vi "Keithley2450_and_2410_plus_lockin.vi"() -> ()   [LabVIEW 2024]
uses:
  <vilib>/Analysis/1siggen.llb/Ramp Pattern by Delta.vi
  <vilib>/Utility/file.llb/Write Delimited Spreadsheet (string).vi
  <vilib>/Utility/file.llb/Write Delimited Spreadsheet (DBL).vi
  C:/Users/Public/OneDrive/Desktop/Keithley_2450_2470_1_4_0_LV2015_NewReadme2_2450-LV2015-1.4.0/Keithley 2450/Keithley 2450.lvlib
  <vilib>/Analysis/NI_AALBase.lvlib
  archive/Keithley 24XX/Keithley 24XX.lvlib
panel:
  out "voltage 2410":dbl format="%0.2f"
  out "Current set voltage 2410":dbl
  in  "V stepsize 2410":dbl
  in  "start V 2410":dbl
  in  "End V 2410":dbl
  out "standard deviation current measured 2450":dbl format="%0.5e"
  out "mean current measured 2450":dbl format="%0.5e"
  out "standard deviation current measured 2410":dbl format="%0.5e"
  out "mean current measured 2410":dbl format="%0.5e"
  in  "Compliance  Level 2410":dbl=1e-06
  in  "VISA resource name 2410":refnum<visa-resource-name>="GPIB0::24::INSTR"
  in  "Serial Configuration":T1={"Baud Rate"=9600, "Parity"=0, "Data Bits"=8, "Stop Bits"=10, "Flow Control"=0} {"Flow Control" items=["None", "XON/XOFF", "RTS/CTS", "XON/XOFF & RTS/CTS", "DTR/DSR", "XON/XOFF & DTR/DSR"]; "Stop Bits" items=["1.0"=10, "1.5"=15, "2.0"=20]; "Data Bits" items=["7"=7, "8"=8]; "Parity" items=["None", "Odd", "Even", "Mark", "Space"]; "Baud Rate" items=["300"=300, "600"=600, "1200"=1200, "2400"=2400, "4800"=4800, "9600"=9600, "19200"=19200]}
  in  "Wait for Current Meas":u32=100
  in  "Number of Current Meas":u32=100
  in  "Loop?":bool=TRUE
  out "Current set voltage 2450":dbl
  in  "V stepsize 2450":dbl
  in  "start V 2450":dbl
  in  "End V 2450":dbl
  in  "Wait for lock in meas (ms)":i32=2000
  in  "File Path":path=path "C:/Users/Public/OneDrive/Desktop/test.txt"
  out "错误输出":errorcluster
  out "Channel AWaveform Chart":dbl[](graph)
  in  "Channel A Waveform Display":string(combo)="A-R"
  in  "Channel B Waveform Display":string(combo)="Channel_B_Rh1"
  out "Channel B Waveform Chart":dbl[](graph)
  out "AUX-ADC4 (V)":sgl format="%.3f"
  out "AUX-ADC3 (V)":sgl format="%.3f"
  out "AUX-ADC1 (V)":sgl format="%.3f"
  out "AUX-ADC2 (V)":sgl format="%.3f"
  out "R":sgl caption="R (Vrms)" format="%.3p"
  out "X":sgl caption="X (Vrms)" format="%.3p"
  out "Y":sgl caption="Y (Vrms)" format="%.3p"
  out "θ (°)":sgl caption="θ (deg)" format="%.2f"
  out "频率 (Hz)":sgl caption="Freq (Hz)" format="%#.3f"
  out "噪声":sgl caption="Noise(Vrms)" format="%.3p"
  out "Rh1":sgl caption="Rh1 (Vrms)" format="%.3p"
  out "θh1 (°)":sgl caption="θh1 (deg)" format="%.2f"
  out "Xh1":sgl caption="Xh1 (Vrms)" format="%.3p"
  out "Yh1":sgl caption="Yh1 (Vrms)" format="%.3p"
  out "X 2":sgl caption="X (Vrms)" format="%.3p"
  out "Y 2":sgl caption="Y (Vrms)" format="%.3p"
  out "R 2":sgl caption="R (Vrms)" format="%.3p"
  out "θ (°) 2":sgl caption="θ (deg)" format="%.2f"
  out "频率 (Hz) 2":sgl caption="Freq (Hz)" format="%#.3f"
  out "噪声 2":sgl caption="Noise(Vrms)" format="%.3p"
  out "Xh1 2":sgl caption="Xh1 (Vrms)" format="%.3p"
  out "Yh1 2":sgl caption="Yh1 (Vrms)" format="%.3p"
  out "Rh1 2":sgl caption="Rh1 (Vrms)" format="%.3p"
  out "θh1 (°) 2":sgl caption="θh1 (deg)" format="%.2f"
  in  "A Sensitivity":u16(ring)=20 items=["1 nV/fA", "2 nV/fA", "5 nV/fA", "10 nV/fA", "20 nV/fA", "50 nV/fA", "100 nV/fA", "200 nV/fA", "500 nV/fA", "1 uV/pA", "2 uV/pA", "5 uV/pA", "10 uV/pA", "20 uV/pA", "50 uV/pA", "100 uV/pA", "200 uV/pA", "500 uV/pA", "1 mV/nA", "2 mV/nA", "5 mV/nA", "10 mV/nA", "20 mV/nA", "50 mV/nA", "100 mV/nA", "200 mV/nA", "500 mV/nA", "1 V/uA"]
  in  "B Sensitivity":u16(ring)=17 items=["1 nV/fA", "2 nV/fA", "5 nV/fA", "10 nV/fA", "20 nV/fA", "50 nV/fA", "100 nV/fA", "200 nV/fA", "500 nV/fA", "1 uV/pA", "2 uV/pA", "5 uV/pA", "10 uV/pA", "20 uV/pA", "50 uV/pA", "100 uV/pA", "200 uV/pA", "500 uV/pA", "1 mV/nA", "2 mV/nA", "5 mV/nA", "10 mV/nA", "20 mV/nA", "50 mV/nA", "100 mV/nA", "200 mV/nA", "500 mV/nA", "1 V/uA"]
  out "序列号":string
  in  "Num Lock in Points":i32=100
  in  "OE1022D":refnum<visa-resource-name>="COM6"
  in  "Current Compliance Limit (0.1) 2450":dbl=5e-08
  in  "VISA resource name 2450":refnum<visa-resource-name>="GPIB0::18::INSTR"
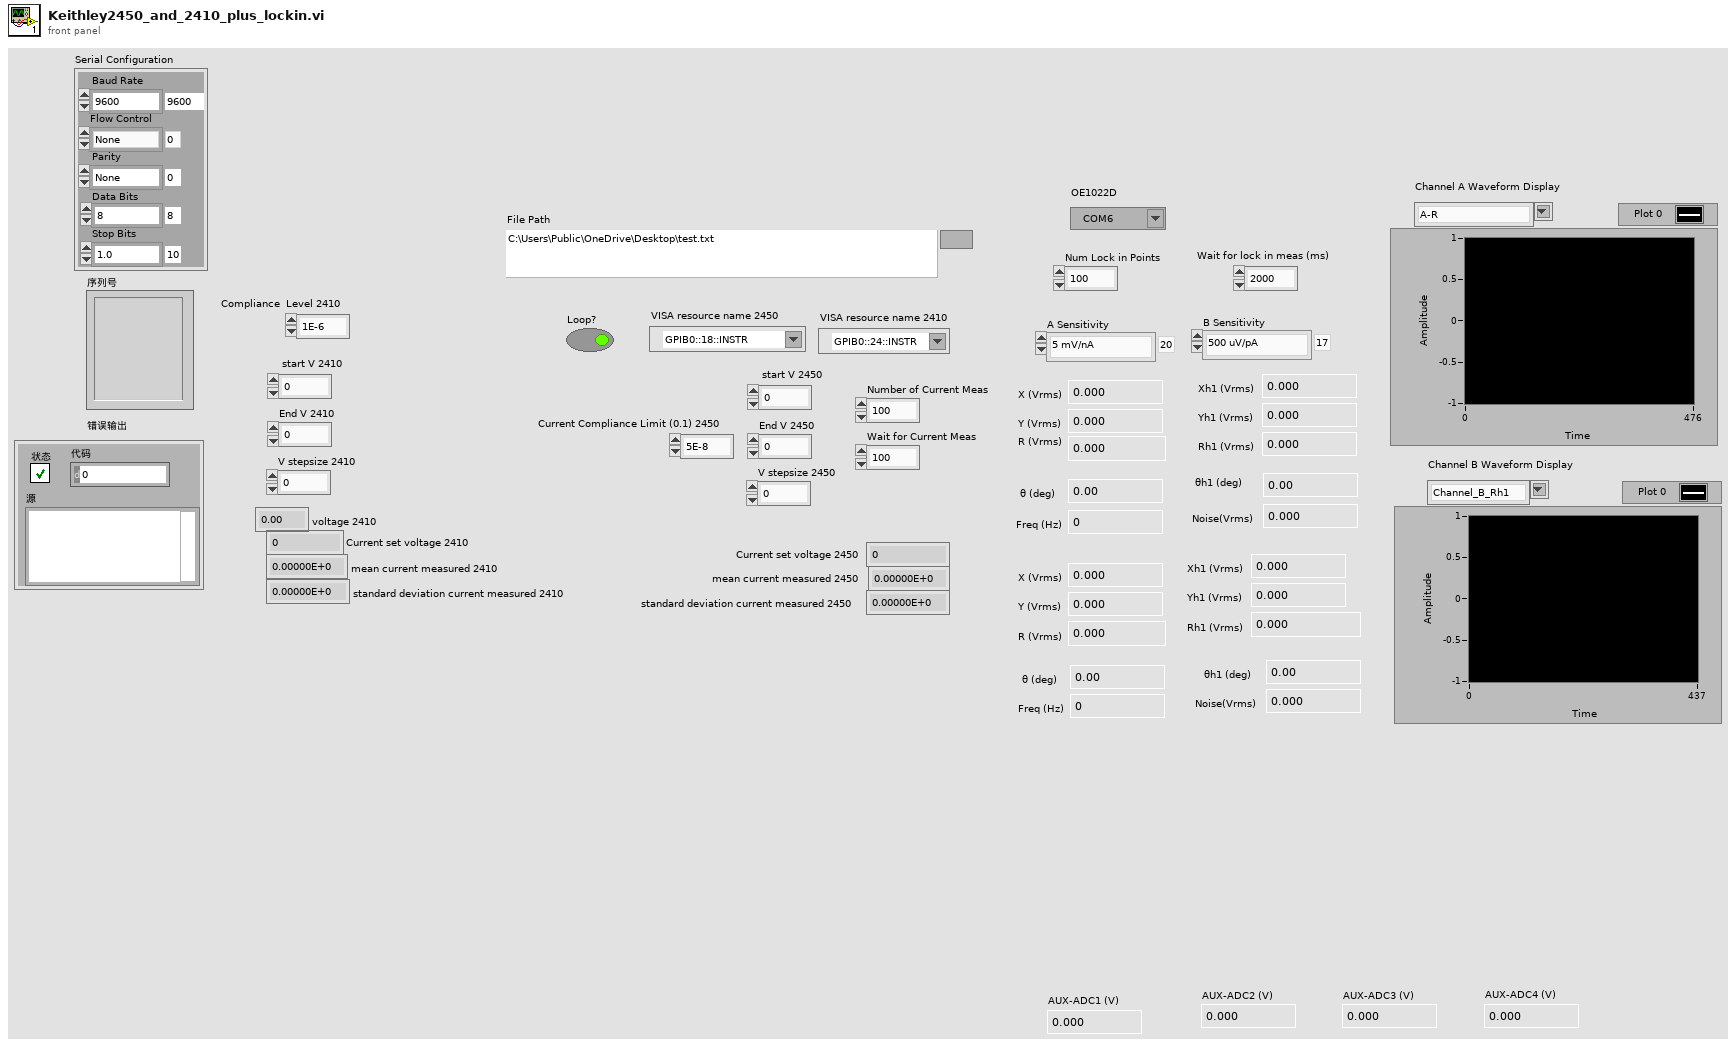
[diagram p1: front panel]
types:
  T1 = cluster{"Baud Rate":u32, "Parity":u16, "Data Bits":u16, "Stop Bits":u16, "Flow Control":u16}
  T2 = cluster{"AD1":dbl[], "AD2":dbl[], "AD3":dbl[], "AD4":dbl[]}
  T3 = cluster{"XB":dbl[], "YB":dbl[], "FrequencyB":dbl[], "NoiseB":dbl[], "Xh1B":dbl[], "Yh1B":dbl[], "Xh2B":dbl[], "Yh2B":dbl[], "Xh2B":dbl[]}
  T4 = cluster{"XA":dbl[], "YA":dbl[], "FrequencyA":dbl[], "NoiseA":dbl[], "Xh1A":dbl[], "Yh1A":dbl[], "Xh2A":dbl[], "Yh2A":dbl[]}
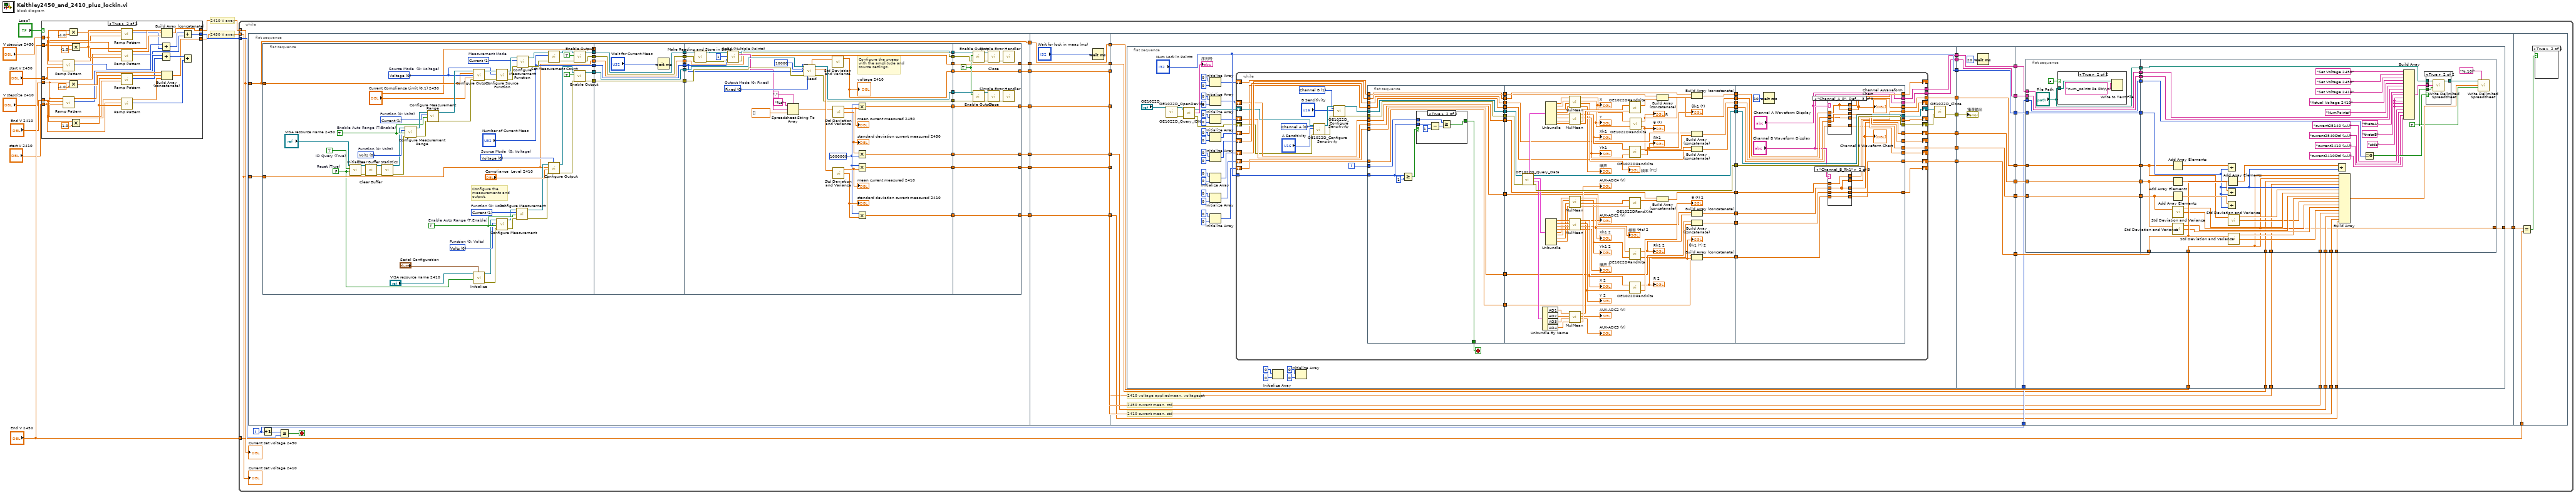
[diagram p0: block diagram]
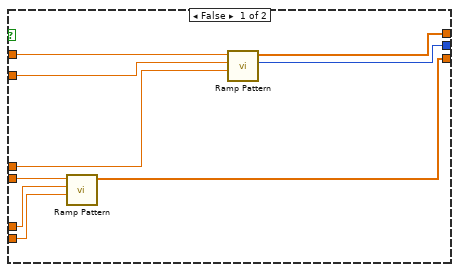
[diagram p2: hidden frame]
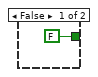
[diagram p3: hidden frame]
diagram:
  # "2410 V array"
  # "2450 V array"
  n1 = case shown="True" "Loop?" {
    tunnel: [w16 w43] -> w10
    tunnel: [w15 w38] -> w9
    tunnel: "V stepsize 2450" -> [w17 w37]
    tunnel: "start V 2450" -> [w18 w36]
    tunnel: "End V 2450" -> [w19 w35]
    tunnel: "End V 2410" -> [w14 w23]
    tunnel: "V stepsize 2410" -> [w12 w21]
    tunnel: "start V 2410" -> [w13 w22]
    tunnel: [w11 w20] -> w1
    frame False {
      n2 = call-poly <vilib>:"Ramp Pattern.vi"("start"=w13, "end"=w14, "delta"=w12) -> ("Ramp Pattern"=w11:dbl[])  [unwired: 6 in, 2 out]
      n3 = call-poly <vilib>:"Ramp Pattern.vi"("start"=w18, "end"=w19, "delta"=w17) -> ("samples"=w15:i32, "Ramp Pattern"=w16:dbl[])  [unwired: 6 in, 1 out]
    }
    frame True {
      n4 = call-poly <vilib>:"Ramp Pattern.vi"("start"=w36, "end"=w35, "delta"=w37) -> ("samples"=w42:i32, "Ramp Pattern"=w46:dbl[])  [unwired: 6 in, 1 out]
      n5 = call-poly <vilib>:"Ramp Pattern.vi"("start"=w22, "end"=w23, "delta"=w21) -> ("samples"=w27:i32, "Ramp Pattern"=w30:dbl[])  [unwired: 6 in, 1 out]
      n6 = Multiply(x=w37, y=-1.0) -> (x*y=w48:dbl)
      n7 = Multiply(x=w21, y=-1.0) -> (x*y=w32:dbl)
      n8 = Multiply(x=w35, y=-1.0) -> (x*y=w47:dbl)
      n9 = Multiply(x=w23, y=-1.0) -> (x*y=w31:dbl)
      n10 = call-poly <vilib>:"Ramp Pattern.vi"("start"=w35, "end"=w47, "delta"=w48) -> ("samples"=w41:i32, "Ramp Pattern"=w45:dbl[])  [unwired: 6 in, 1 out]
      n11 = call-poly <vilib>:"Ramp Pattern.vi"("start"=w47, "end"=w36, "delta"=w37) -> ("samples"=w40:i32, "Ramp Pattern"=w44:dbl[])  [unwired: 6 in, 1 out]
      n12 = call-poly <vilib>:"Ramp Pattern.vi"("start"=w23, "end"=w31, "delta"=w32) -> ("samples"=w26:i32, "Ramp Pattern"=w29:dbl[])  [unwired: 6 in, 1 out]
      n13 = call-poly <vilib>:"Ramp Pattern.vi"("start"=w31, "end"=w22, "delta"=w21) -> ("samples"=w25:i32, "Ramp Pattern"=w28:dbl[])  [unwired: 6 in, 1 out]
      n14 = Add(x=w42, y=w41) -> (x+y=w39:i32)
      n15 = Add(x=w27, y=w26) -> (x+y=w24:i32)
      n16 = Build Array (concatenate)(w46, w45, w44) -> (w43:dbl[])
      n17 = Build Array (concatenate)(w30, w29, w28) -> (w20:dbl[])
      n18 = Add(x=w39, y=w40) -> (x+y=w38:i32)
      n19 = Add(x=w24, y=w25) -> ()  [unwired: 1 out]
    }
  }
  n20 = while {
    tunnel: w10 -> [w70] mode=indexing
    tunnel: w9 -> [w72]
    tunnel: "End V 2450" -> [w64]
    tunnel: w1 -> [w51] mode=indexing
    i -> [w66]
    stop <- w71 stop-if-true
    n21 = flat-sequence {
      tunnel: w70 -> [w103]
      tunnel: [w103] -> w68
      tunnel: [w85] -> w62
      tunnel: [w84] -> w60
      tunnel: [w83] -> w58
      tunnel: [w82] -> w56
      tunnel: [w80] -> w54
      tunnel: [w76] -> w53
      tunnel: w51 -> [w75]
      tunnel: w68 -> [w217]
      tunnel: [w217] -> w67
      tunnel: [w216] -> w63
      tunnel: w62 -> [w216]
      tunnel: [w215] -> w61
      tunnel: w60 -> [w215]
      tunnel: [w214] -> w59
      tunnel: w58 -> [w214]
      tunnel: [w213] -> w57
      tunnel: w56 -> [w213]
      tunnel: [w212] -> w55
      tunnel: w54 -> [w212]
      tunnel: w53 -> [w211]
      tunnel: [w211] -> w52
      tunnel: w67 -> [w227]
      tunnel: w66 -> [w226]
      tunnel: [w225] -> w65
      tunnel: w63 -> [w224]
      tunnel: w61 -> [w223]
      tunnel: w59 -> [w222]
      tunnel: w57 -> [w221]
      tunnel: w55 -> [w220]
      tunnel: w52 -> [w219]
      tunnel: w65 -> [w579]
      tunnel: w64 -> [w580]
      frame #0 {
        n22 = flat-sequence {
          tunnel: w103 -> [w138]
          tunnel: [w137] -> w102
          tunnel: ["Current Compliance Limit (0.1) 2450"] -> w100
          tunnel: [w135] -> w99
          tunnel: [w121] -> w97
          tunnel: [w120] -> w96
          tunnel: ["Number of Current Meas"] -> w90
          tunnel: [w111] -> w78
          tunnel: w75 -> [w111]
          tunnel: w102 -> [w161]
          tunnel: [w161] -> w101
          tunnel: w100 -> [_]
          tunnel: w99 -> [w160]
          tunnel: [w160] -> w98
          tunnel: w97 -> [w158]
          tunnel: w96 -> [w157]
          tunnel: [w158] -> w95
          tunnel: [w157] -> w94
          tunnel: [w156] -> w91
          tunnel: w90 -> [w156]
          tunnel: [w155] -> w79
          tunnel: w78 -> [w155]
          tunnel: w101 -> [w186]
          tunnel: w98 -> [w174]
          tunnel: w95 -> [w190]
          tunnel: w94 -> [w189]
          tunnel: [w188] -> w93
          tunnel: [w187] -> w92
          tunnel: w91 -> [w183]
          tunnel: [w177] -> w89
          tunnel: [w176] -> w88
          tunnel: [w164] -> w87
          tunnel: [w166] -> w86
          tunnel: [w171] -> w81
          tunnel: w79 -> [w172]
          tunnel: [w172] -> w77
          tunnel: [w170] -> w74
          tunnel: [w167] -> w73
          tunnel: w93 -> [w210]
          tunnel: w92 -> [w209]
          tunnel: w89 -> [w208]
          tunnel: w88 -> [w207]
          tunnel: w87 -> [w202]
          tunnel: w86 -> [w201]
          tunnel: [w202] -> w85
          tunnel: [w201] -> w84
          tunnel: [w200] -> w83
          tunnel: [w199] -> w82
          tunnel: [w198] -> w80
          tunnel: w81 -> [w198]
          tunnel: w77 -> [w197]
          tunnel: [w197] -> w76
          tunnel: w74 -> [w199]
          tunnel: w73 -> [w200]
          frame #0 {
            w117 = u16 0 items=["Voltage", "Current"]  # Source Mode  (0: Voltage)
            w134 = TRUE  # Enable Auto Range (T:Enable)
            w130 = u16 1 items=["Volts", "Current", "Resistance"]  # Function (0: Volts)
            w129 = u16 0 items=["Volts", "Current", "Resistance"]  # Function (0: Volts)
            w139 = u16 0 items=["Voltage", "Current"]  # Source Mode  (0: Voltage)
            w140 = u16 1 items=["Volts", "Current", "Auto Resistance", "Manual Resistance", "Digitize Voltage", "Digitize Current"]  # Measurement Mode
            w144 = TRUE  # Enable Auto Range (T:Enable)
            w142 = u16 1 items=["Volts", "Current", "Resistance"]  # Function (0: Volts)
            w143 = u16 0 items=["Volts", "Current", "Resistance"]  # Function (0: Volts)
            w110 = FALSE  # Reset (True)
            w145 = TRUE  # ID Query (True)
            # "Configure the measurements and output."
            n23 = call "Initialize.vi"("Reset (True)"=w110, "ID Query (True)"=w145, "VISA resource name"="VISA resource name 2450") -> ("error out"=w108:errorcluster, "VISA resource name out"=w109:refnum<visa-resource-name>)  [unwired: 7 in]
            n24 = call "Clear Buffer.vi"("VISA resource name"=w109, "error in (no error)"=w108) -> ("VISA resource name out"=w107:refnum<visa-resource-name>, "error out"=w104:errorcluster)  [unwired: 12 in]
            n25 = call "Clear Buffer Statistics.vi"("VISA resource name"=w107, "error in (no error)"=w104) -> ("VISA resource name out"=w106:refnum<visa-resource-name>, "error out"=w105:errorcluster)  [unwired: 12 in]
            n26 = call "Configure Measurement Range.vi"("error in (no error)"=w105, "Enable Auto Range (T:Enable)"=w144, "Function (0: Volts)"=w143, "VISA resource name"=w106) -> ("error out"=w147:errorcluster, "VISA resource name out"=w146:refnum<visa-resource-name>)  [unwired: 6 in]
            n27 = call "Configure Measurement Range.vi"("error in (no error)"=w147, "Enable Auto Range (T:Enable)"=w144, "Function (0: Volts)"=w142, "VISA resource name"=w146) -> ("error out"=w152:errorcluster, "VISA resource name out"=w153:refnum<visa-resource-name>)  [unwired: 6 in]
            n28 = call "Configure Output.vi"("VISA resource name"=w153, "Source Level (0)"=w138, "Source Mode  (0: Voltage)"=w139, "Source Limit Level (0.1)"="Current Compliance Limit (0.1) 2450", "error in (no error)"=w152) -> ("VISA resource name out"=w148:refnum<visa-resource-name>, "error out"=w149:errorcluster)  [unwired: 9 in]
            n29 = call "Initialize.vi"("Serial Configuration"="Serial Configuration", "Reset (True)"=w110, "VISA resource name"="VISA resource name 2410") -> ("error out"=w123:errorcluster, "VISA resource name out"=w122:refnum<visa-resource-name>)  [unwired: 7 in]
            n30 = call "Configure Source Function.vi"("error in (no error)"=w149, "Function (0: Volts)"=w139, "VISA resource name"=w148) -> ("error out"=w150:errorcluster, "VISA resource name out"=w151:refnum<visa-resource-name>)  [unwired: 7 in]
            n31 = call "Configure Measurement.vi"("error in (no error)"=w123, "Enable Auto Range (T:Enable)"=w134, "Function (0: Volts)"=w129, "VISA resource name"=w122) -> ("error out"=w124:errorcluster, "VISA resource name out"=w125:refnum<visa-resource-name>)  [unwired: 6 in]
            n32 = call "Configure Measurement.vi"("error in (no error)"=w124, "Enable Auto Range (T:Enable)"=w134, "Function (0: Volts)"=w130, "VISA resource name"=w125) -> ("error out"=w118:errorcluster, "VISA resource name out"=w119:refnum<visa-resource-name>)  [unwired: 6 in]
            n33 = call "Configure Measurement Function.vi"("error in (no error)"=w150, "Function (0: Volts)"=w140, "VISA resource name"=w151) -> ("error out"=w115:errorcluster, "VISA resource name out"=w116:refnum<visa-resource-name>)  [unwired: 7 in]
            n34 = call "Set Measurement Count.vi"("error in (no error)"=w115, "Measurement Count"="Number of Current Meas", "VISA resource name"=w116) -> ("error out"=w114:errorcluster, "VISA resource name out"=w113:refnum<visa-resource-name>)  [unwired: 7 in]
            n35 = call "Configure Output.vi"("Source Mode  (0: Voltage)"=w117, "error in (no error)"=w118, "Compliance  Level (0.1)"="Compliance  Level 2410", "Output Level (0)"=w111, "VISA resource name"=w119) -> ("error out"=w133:errorcluster, "VISA resource name out"=w132:refnum<visa-resource-name>)  [unwired: 5 in]
            n36 = call "Enable Output.vi"("error in (no error)"=w114, "Enable Output (T: Enable)"=TRUE, "VISA resource name"=w113) -> ("error out"=w135:errorcluster, "VISA resource name out"=w137:refnum<visa-resource-name>)  [unwired: 7 in]
            n37 = call "Enable Output.vi"("error in (no error)"=w133, "Enable Output (T: Enable)"=TRUE, "VISA resource name"=w132) -> ("error out"=w120:errorcluster, "VISA resource name out"=w121:refnum<visa-resource-name>)  [unwired: 7 in]
          }
          frame #1 {
            n38 = Wait (ms)(milliseconds to wait="Wait for Current Meas") -> ()  [unwired: 1 out]
          }
          frame #2 {
            w162 = 1000000 ("Timeout (10000 ms)")
            w192 = u16 0 items=["Fixed", "Sweep", "List"]  # Output Mode (0: Fixed)
            # "Configure the sweep with the amplitude and source settings."
            n39 = call "Make Reading and Store in Buffer.vi"("VISA resource name"=w186, "error in (no error)"=w174) -> ("VISA resource name out"=w184:refnum<visa-resource-name>, "error out"=w185:errorcluster)  [unwired: 12 in]
            n40 = call "Read (Multiple Points).vi"("VISA resource name"=w184, "Start Index (1)"=u32 1, "End Index (1)"=w183, "error in (no error)"=w185) -> ("VISA resource name out"=w177:refnum<visa-resource-name>, "Data out"=w178:string, "error out"=w176:errorcluster)  [unwired: 9 in]
            n41 = Spreadsheet String To Array(delimiter (Tab)=",", format string="%s", spreadsheet string=w178, array type (2D Dbl)=dbl[] []) -> (array=w175:dbl[])
            n42 = call-poly "Read.vi"("VISA resource name"=w190, "Sample Count (1)"=w183, "Timeout (10000 ms)"=10000, "error in (no error)"=w189, "Output Mode (0: Fixed)"=w192) -> ("Voltage"=w173:sgl[], "VISA resource name out"=w187:refnum<visa-resource-name>, "Current"=w191:sgl[], "error out"=w188:errorcluster)  [unwired: 4 in, 3 out]
            n43 = call <vilib>:"Std Deviation and Variance.vi"("X"=w173) -> ("mean"=w171:dbl)  [unwired: 1 in, 2 out]
            "voltage 2410" <- w171
            n44 = call <vilib>:"Std Deviation and Variance.vi"("X"=w175) -> ("mean"=w163:dbl, "standard deviation"=w165:dbl)  [unwired: 1 in, 1 out]
            "mean current measured 2450" <- w163
            "standard deviation current measured 2450" <- w165
            n45 = call <vilib>:"Std Deviation and Variance.vi"("X"=w191) -> ("mean"=w168:dbl, "standard deviation"=w169:dbl)  [unwired: 1 in, 1 out]
            "mean current measured 2410" <- w168
            "standard deviation current measured 2410" <- w169
            n46 = Multiply(x=w162, y=w163) -> (x*y=w164:dbl)
            n47 = Multiply(x=w165, y=w162) -> (x*y=w166:dbl)
            n48 = Multiply(x=w162, y=w168) -> (x*y=w167:dbl)
            n49 = Multiply(x=w162, y=w169) -> (x*y=w170:dbl)
          }
          frame #3 {
            w206 = TRUE ("Enable Output (T: Enable)")
            n50 = call "Enable Output.vi"("error in (no error)"=w207, "Enable Output (T: Enable)"=w206, "VISA resource name"=w208) -> ("error out"=w204:errorcluster, "VISA resource name out"=w205:refnum<visa-resource-name>)  [unwired: 7 in]
            n51 = call "Enable Output.vi"("error in (no error)"=w210, "Enable Output (T: Enable)"=w206, "VISA resource name"=w209) -> ("error out"=w195:errorcluster, "VISA resource name out"=w196:refnum<visa-resource-name>)  [unwired: 7 in]
            n52 = call "Close.vi"("error in (no error)"=w204, "VISA resource name"=w205) -> ("error out"=w203:errorcluster)  [unwired: 9 in]
            n53 = call "Close.vi"("error in (no error)"=w195, "VISA resource name"=w196) -> ("error out"=w194:errorcluster)  [unwired: 9 in]
            n54 = call <vilib>:"Simple Error Handler.vi"("error in (no error)"=w203) -> ()  [unwired: 4 in, 5 out]
            n55 = call <vilib>:"Simple Error Handler.vi"("error in (no error)"=w194) -> ()  [unwired: 4 in, 5 out]
          }
        }
      }
      frame #1 {
        n56 = Wait (ms)(milliseconds to wait="Wait for lock in meas (ms)") -> ()  [unwired: 1 out]
      }
      frame #2 {
        # "2410 voltage appliedmean, voltageset"
        # "2410 current mean, std"
        # "2450 current mean, std"
        n57 = flat-sequence {
          tunnel: [w263] -> w242
          tunnel: [w262] -> w241
          tunnel: ["Num Lock in Points"] -> w240
          tunnel: [w257] -> w239
          tunnel: [w261] -> w238
          tunnel: [w260] -> w237
          tunnel: [w247] -> w236
          tunnel: [w248] -> w235
          tunnel: w242 -> [w491]
          tunnel: [w491] -> w234
          tunnel: w241 -> [w490]
          tunnel: [w490] -> w233
          tunnel: w240 -> [w489]
          tunnel: [w489] -> w232
          tunnel: w239 -> [w487]
          tunnel: [w486] -> w231
          tunnel: w238 -> [w486]
          tunnel: w237 -> [w485]
          tunnel: [w485] -> w230
          tunnel: [w484] -> w229
          tunnel: w236 -> [w484]
          tunnel: w235 -> [w483]
          tunnel: [w483] -> w228
          tunnel: w234 -> [w511]
          tunnel: w233 -> [w510]
          tunnel: w232 -> [w509]
          tunnel: w231 -> [w507]
          tunnel: w230 -> [w506]
          tunnel: w229 -> [w504]
          tunnel: w228 -> [w502]
          tunnel: w227 -> [w501]
          tunnel: w226 -> [w499]
          tunnel: [w498] -> w225
          tunnel: w224 -> [w497]
          tunnel: w223 -> [w496]
          tunnel: w222 -> [w495]
          tunnel: w221 -> [w494]
          tunnel: w220 -> [w492]
          tunnel: w219 -> [w493]
          frame #0 {
            n58 = call "OE1022D_OpenDevice.vi"("VISA resource name"="OE1022D") -> ("VISA资源名称输出"=w285:refnum<visa-resource-name>, "错误输出"=w284:errorcluster)  [unwired: 17 in]
            n59 = call "OE1022D_Query_IDN.vi"("错误输入（无错误）"=w284, "VISA resource name"=w285) -> ("错误输出"=w255:errorcluster, "序列号"=→"序列号":string, "VISA resource name out"=w256:refnum<visa-resource-name>)  [unwired: 1 in]
            n60 = Initialize Array(0, 0) -> (w281:i32[])
            n61 = Initialize Array(0, 0) -> (w265:i32[])
            n62 = Initialize Array(0, 0) -> (w264:i32[])
            n63 = Initialize Array(0, 0) -> (w250:i32[])
            n64 = Initialize Array(0, 0) -> (w270:i32[])
            n65 = Initialize Array(0, 0) -> (w271:i32[])
            n66 = Initialize Array(0, 0) -> (w249:i32[])
            n67 = Initialize Array(0, 0) -> (w276:i32[])
            n68 = while {
              shift-right: [w338] -> _
              shift-left: w281 -> [w337]
              shift-right: [w335] -> _
              shift-left: w276 -> [w334]
              tunnel: "Num Lock in Points" -> [w327]
              shift-right: [w315] -> _
              shift-left: w270 -> [w317]
              shift-right: [w311] -> _
              shift-left: w271 -> [w314]
              shift-right: [w304] -> _
              shift-left: w264 -> [w310]
              shift-right: [w303] -> _
              shift-left: w265 -> [w309]
              tunnel: [w302] -> w263
              tunnel: [w301] -> w262
              tunnel: [w300] -> w261
              tunnel: [w299] -> w260
              shift-right: [w298] -> w259
              shift-left: w255 -> [w295]
              shift-right: [w297] -> w258
              shift-left: w256 -> [w296]
              shift-right: [w287] -> w247
              shift-left: w250 -> [w291]
              shift-right: [w288] -> w248
              shift-left: w249 -> [w289]
              i -> [w329]
              stop <- w328 stop-if-true
              w320 = u8 1 items=["Channel A", "Channel B"] ("OE1022D A/B")
              w326 = u8 0 items=["Channel A", "Channel B"] ("OE1022D A/B")
              n69 = call "OE1022D_Configure Sensitivity.vi"("VISA resource name"=w296, "OE1022D A/B"=w326, "Sensitivity"="A Sensitivity", "error in (no error)"=w295) -> ("VISA resource name out"=w321:refnum<visa-resource-name>, "error out"=w322:errorcluster)  [unwired: 14 in]
              n70 = call "OE1022D_Configure Sensitivity.vi"("VISA resource name"=w321, "OE1022D A/B"=w320, "Sensitivity"="B Sensitivity", "error in (no error)"=w322) -> ("VISA resource name out"=w324:refnum<visa-resource-name>, "error out"=w323:errorcluster)  [unwired: 14 in]
              n71 = flat-sequence {
                tunnel: w334 -> [w353]
                tunnel: w337 -> [w354]
                tunnel: w324 -> [w355]
                tunnel: w323 -> [w356]
                tunnel: [w356] -> w333
                tunnel: [w355] -> w332
                tunnel: [w354] -> w331
                tunnel: [w353] -> w330
                tunnel: w329 -> [w352]
                tunnel: [w351] -> w328
                tunnel: w327 -> [w349]
                tunnel: [w347] -> w318
                tunnel: w317 -> [w347]
                tunnel: w314 -> [w346]
                tunnel: [w346] -> w313
                tunnel: w310 -> [w345]
                tunnel: w309 -> [w344]
                tunnel: [w345] -> w308
                tunnel: [w344] -> w307
                tunnel: [w343] -> w292
                tunnel: w291 -> [w343]
                tunnel: [w342] -> w290
                tunnel: w289 -> [w342]
                tunnel: [w433] -> w341
                tunnel: [w432] -> w340
                tunnel: [w385] -> w339
                tunnel: [w381] -> w336
                tunnel: w333 -> [w435]
                tunnel: w332 -> [w434]
                tunnel: w331 -> [w386]
                tunnel: w330 -> [w383]
                tunnel: w318 -> [w379]
                tunnel: [w378] -> w316
                tunnel: w313 -> [w376]
                tunnel: [w375] -> w312
                tunnel: w308 -> [w371]
                tunnel: w307 -> [w372]
                tunnel: [w370] -> w306
                tunnel: [w369] -> w305
                tunnel: [w365] -> w294
                tunnel: [w367] -> w293
                tunnel: w292 -> [w364]
                tunnel: w290 -> [w363]
                tunnel: w341 -> [w456]
                tunnel: w340 -> [w457]
                tunnel: w339 -> [w455]
                tunnel: [w453] -> w338
                tunnel: w336 -> [w449]
                tunnel: [w448] -> w335
                tunnel: [w457] -> w297
                tunnel: [w456] -> w298
                tunnel: w316 -> [w454]
                tunnel: [w452] -> w315
                tunnel: w312 -> [w451]
                tunnel: [w450] -> w311
                tunnel: w306 -> [w444]
                tunnel: w305 -> [w447]
                tunnel: [w446] -> w304
                tunnel: [w445] -> w303
                tunnel: [w443] -> w302
                tunnel: [w442] -> w301
                tunnel: ["Channel A Waveform Display"] -> w300
                tunnel: ["Channel B Waveform Display"] -> w299
                tunnel: w294 -> [w438]
                tunnel: [w437] -> w287
                tunnel: [w436] -> w288
                tunnel: w293 -> [w439]
                frame #0 {
                  n72 = Greater Or Equal?(x=w349, y=1) -> (x >= y?=w348:bool)
                  n73 = case shown="True" w348 {
                    tunnel: w352 -> [_ w362]
                    tunnel: [FALSE w361] -> w351
                    tunnel: w349 -> [_ w358]
                    frame False {
                    }
                    frame True {
                      n74 = Subtract(x=w358, y=1) -> (x-y=w359:i32)
                      n75 = Greater Or Equal?(x=w362, y=w359) -> (x >= y?=w361:bool)
                    }
                  }
                }
                frame #1 {
                  n76 = call "OE1022D_Query_Data.vi"("错误输入（无错误）"=w435, "VISA resource name"=w434) -> ("error out"=w433:errorcluster, "输出簇ADC"=w389:T2, "输出簇B"=w388:T3, "VISA resource name out"=w432:refnum<visa-resource-name>, "输出簇A"=w382:T4)  [unwired: 3 in]
                  n77 = Unbundle By Name(w389) -> ("AD1"=w428:dbl[], "AD2"=w429:dbl[], "AD3"=w430:dbl[], "AD4"=w431:dbl[])
                  n78 = Unbundle(w382) -> ("XA"=w394:dbl[], "YA"=w395:dbl[], "FrequencyA"=w396:dbl[], "NoiseA"=w397:dbl[], "Xh1A"=w402:dbl[], "Yh1A"=w403:dbl[], "Xh2A"=w404:dbl[], "Yh2A"=w405:dbl[])
                  n79 = Unbundle(w388) -> ("XB"=w418:dbl[], "YB"=w417:dbl[], "FrequencyB"=w416:dbl[], "NoiseB"=w415:dbl[], "Xh1B"=w414:dbl[], "Yh1B"=w413:dbl[], "Xh2B"=w412:dbl[], "Yh2B"=w411:dbl[])  [unwired: 1 out]
                  n80 = call "MulMean.vi"("IN 4"=w397, "IN 3"=w396, "IN 2"=w395, "IN 1"=w394) -> ("mean 4"=→"噪声":dbl, "mean 3"=→"频率 (Hz)":dbl, "mean 2"=w400:dbl, "mean 1"=w399:dbl)  [unwired: 4 in]
                  "X" <- w399
                  "Y" <- w400
                  n81 = call "MulMean.vi"("IN 4"=w405, "IN 3"=w404, "IN 2"=w403, "IN 1"=w402) -> ("mean 4"=w410:dbl, "mean 3"=w409:dbl, "mean 2"=w407:dbl, "mean 1"=w406:dbl)  [unwired: 4 in]
                  "Xh1" <- w406
                  "Yh1" <- w407
                  n82 = call "MulMean.vi"("IN 4"=w411, "IN 3"=w412, "IN 2"=w413, "IN 1"=w414) -> ("mean 4"=w427:dbl, "mean 3"=w426:dbl, "mean 2"=w425:dbl, "mean 1"=w424:dbl)  [unwired: 4 in]
                  "Xh1 2" <- w424
                  "Yh1 2" <- w425
                  n83 = call "MulMean.vi"("IN 4"=w415, "IN 3"=w416, "IN 2"=w417, "IN 1"=w418) -> ("mean 4"=→"噪声 2":dbl, "mean 3"=→"频率 (Hz) 2":dbl, "mean 2"=w423:dbl, "mean 1"=w422:dbl)  [unwired: 4 in]
                  "X 2" <- w422
                  "Y 2" <- w423
                  n84 = call "MulMean.vi"("IN 4"=w431, "IN 3"=w430, "IN 2"=w429, "IN 1"=w428) -> ("mean 4"=→"AUX-ADC4 (V)":dbl, "mean 3"=→"AUX-ADC3 (V)":dbl, "mean 2"=→"AUX-ADC2 (V)":dbl, "mean 1"=→"AUX-ADC1 (V)":dbl)  [unwired: 4 in]
                  n85 = call "OE1022DRandXita.vi"("Y"=w410, "X"=w409) -> ("R"=w377:dbl)  [unwired: 1 out]
                  n86 = call "OE1022DRandXita.vi"("Y"=w427, "X"=w426) -> ("R"=w373:dbl)  [unwired: 1 out]
                  n87 = call "OE1022DRandXita.vi"("Y"=w407, "X"=w406) -> ("θ (°)"=→"θh1 (°)":dbl, "R"=w380:dbl)
                  "Rh1" <- w380
                  n88 = call "OE1022DRandXita.vi"("Y"=w425, "X"=w424) -> ("θ (°)"=w368:dbl, "R"=w374:dbl)
                  "Rh1 2" <- w374
                  "θh1 (°) 2" <- w368
                  n89 = call "OE1022DRandXita.vi"("Y"=w423, "X"=w422) -> ("θ (°)"=→"θ (°) 2":dbl, "R"=w384:dbl)
                  "R 2" <- w384
                  n90 = call "OE1022DRandXita.vi"("Y"=w400, "X"=w399) -> ("θ (°)"=w366:dbl, "R"=w387:dbl)
                  "R" <- w387
                  "θ (°)" <- w366
                  n91 = Build Array (concatenate)(w376, w377) -> (w375:dbl[])
                  n92 = Build Array (concatenate)(w372, w373) -> (w369:dbl[])
                  n93 = Build Array (concatenate)(w386, w387) -> (w385:dbl[])
                  n94 = Build Array (concatenate)(w379, w380) -> (w378:dbl[])
                  n95 = Build Array (concatenate)(w364, w366) -> (w365:dbl[])
                  n96 = Build Array (concatenate)(w371, w374) -> (w370:dbl[])
                  n97 = Build Array (concatenate)(w383, w384) -> (w381:dbl[])
                  n98 = Build Array (concatenate)(w363, w368) -> (w367:dbl[])
                }
                frame #2 {
                  n99 = Wait (ms)(milliseconds to wait=10) -> ()  [unwired: 1 out]
                  n100 = case shown="\"Channel_A_R\", Default" "Channel A Waveform Display" {
                    tunnel: w455 -> [w474 w478 w480]
                    tunnel: [w474 w478 w480] -> w453
                    tunnel: w454 -> [w472 w477 w482]
                    tunnel: [w472 w477 w482] -> w452
                    tunnel: w451 -> [w473 w476 w481]
                    tunnel: [w473 w476 w481] -> w450
                    tunnel: [w472 w476 w480] -> w443
                    tunnel: w438 -> [w471 w475 w479]
                    tunnel: [w471 w475 w479] -> w437
                    frame "Channel_A_Rh1" {
                    }
                    frame "Channel_A_Rh2" {
                    }
                    frame "Channel_A_R", Default {
                    }
                  }
                  "Channel AWaveform Chart" <- w443
                  n101 = case shown="\"Channel_B_Rh1\"" "Channel B Waveform Display" {
                    tunnel: [w462 w464 w468] -> w442
                    tunnel: w449 -> [w462 w466 w470]
                    tunnel: [w462 w466 w470] -> w448
                    tunnel: w447 -> [w461 w465 w468]
                    tunnel: [w461 w465 w468] -> w445
                    tunnel: [w460 w464 w469] -> w446
                    tunnel: w444 -> [w460 w464 w469]
                    tunnel: w439 -> [w459 w463 w467]
                    tunnel: [w459 w463 w467] -> w436
                    frame "Channel_B_R", Default {
                    }
                    frame "Channel_B_Rh1" {
                    }
                    frame "Channel_B_Rh2" {
                    }
                  }
                  "Channel B Waveform Chart" <- w442
                }
              }
            }
            n102 = Initialize Array(0, 0) -> ()  [unwired: 1 out]
            n103 = Initialize Array(0, 0) -> ()  [unwired: 1 out]
            n104 = call "OE1022D_Close.vi"("错误输入（无错误）"=w259, "VISA resource name"=w258) -> ("错误输出"=w257:errorcluster)  [unwired: 1 in]
          }
          frame #1 {
            n105 = Wait (ms)(milliseconds to wait=20) -> ()  [unwired: 1 out]
            "错误输出" <- w487
          }
          frame #2 {
            n106 = flat-sequence {
              tunnel: w509 -> [w522]
              tunnel: w510 -> [w523]
              tunnel: w511 -> [w524]
              tunnel: [w524] -> w515
              tunnel: [w523] -> w514
              tunnel: [w522] -> w513
              tunnel: ["File Path"] -> w512
              tunnel: [w519] -> w508
              tunnel: w507 -> [w519]
              tunnel: w506 -> [w518]
              tunnel: [w518] -> w505
              tunnel: w504 -> [w517]
              tunnel: [w517] -> w503
              tunnel: [w516] -> w500
              tunnel: w499 -> [w516]
              tunnel: w515 -> [w554]
              tunnel: w514 -> [w557]
              tunnel: w513 -> [w560]
              tunnel: w512 -> [w567]
              tunnel: w508 -> [w565]
              tunnel: w505 -> [w564]
              tunnel: w503 -> [w555]
              tunnel: w502 -> [w556]
              tunnel: w501 -> [w532]
              tunnel: w500 -> [w542]
              tunnel: [w532] -> w498
              tunnel: w497 -> [w540]
              tunnel: w496 -> [w539]
              tunnel: w495 -> [w538]
              tunnel: w494 -> [w537]
              tunnel: w493 -> [w534]
              tunnel: w492 -> [w533]
              frame #0 {
                n107 = case shown="True" FALSE {
                  tunnel: "File Path" -> [_ w526]
                  frame False {
                  }
                  frame True {
                    n108 = Write to Text File(file (use dialog)=w526, text="num_points Ra Rb\r\n") -> ()  [unwired: 2 in, 3 out]
                  }
                }
              }
              frame #1 {
                w545 = "stds"
                w566 = TRUE
                n109 = Add Array Elements(numeric array=w554) -> (sum=w571:dbl)
                n110 = Add Array Elements(numeric array=w555) -> (sum=w562:dbl)
                n111 = Add Array Elements(numeric array=w557) -> (sum=w569:dbl)
                n112 = call <vilib>:"Std Deviation and Variance.vi"("X"=w557) -> ("mean"=w552:dbl, "standard deviation"=w546:dbl)  [unwired: 1 in, 1 out]
                n113 = call <vilib>:"Std Deviation and Variance.vi"("X"=w555) -> ("mean"=w551:dbl, "standard deviation"=w548:dbl)  [unwired: 1 in, 1 out]
                n114 = Divide(x=w571, y=w560) -> ()  [unwired: 1 out]
                n115 = Divide(x=w562, y=w560) -> ()  [unwired: 1 out]
                n116 = Divide(x=w569, y=w560) -> ()  [unwired: 1 out]
                n117 = Add Array Elements(numeric array=w556) -> (sum=w561:dbl)
                n118 = call <vilib>:"Std Deviation and Variance.vi"("X"=w554) -> ("mean"=w553:dbl, "standard deviation"=w547:dbl)  [unwired: 1 in, 1 out]
                n119 = call <vilib>:"Std Deviation and Variance.vi"("X"=w556) -> ("mean"=w550:dbl, "standard deviation"=w549:dbl)  [unwired: 1 in, 1 out]
                n120 = Divide(x=w561, y=w560) -> ()  [unwired: 1 out]
                n121 = Build Array(w532, w532, w534, w533, w560, w553, w552, w551, w550, w547, w546, w548, w549, w540, w539, w538, w537) -> (w570:dbl[])
                n122 = Equal To 0?(x=w542) -> (x = 0?=w541:bool)
                n123 = Build Array("Set Voltage 2450", "Set Voltage 2450", "Set Voltage 2410", "Actual Voltage 2410", "NumPoints", w565, w564, "thetaA", "thetaB", w545, w545, w545, w545, "current25140 (uA)", "current2540Std (uA)", "current2410 (uA)", "current2410Std (uA)") -> (w563:string[])
                n124 = case shown="True" w541 {
                  tunnel: [w573 w577] -> w568
                  tunnel: w567 -> [w573 w576]
                  tunnel: w566 -> [_ w575]
                  tunnel: w563 -> [_ w574]
                  frame False {
                  }
                  frame True {
                    n125 = call-poly <vilib>:"Write Delimited Spreadsheet.vi"("file path (dialog if empty)"=w576, "1D data"=w574, "append to file? (new file:F)"=w575) -> ("new file path (Not A Path if cancelled)"=w577:path)  [unwired: 11 in, 1 out]
                  }
                }
                n126 = call-poly <vilib>:"Write Delimited Spreadsheet.vi"("file path (dialog if empty)"=w568, "format (%.3f)"="%.10f", "1D data"=w570, "append to file? (new file:F)"=w566) -> ()  [unwired: 10 in, 2 out]
              }
            }
          }
        }
      }
      frame #3 {
        n127 = Equal?(x=w579, y=w580) -> (x = y?=w578:bool)
        n128 = case shown="True" w578 {
          frame False {
          }
          frame True {
          }
        }
      }
    }
    n129 = Increment(x=w66) -> (x+1=w69:i32)
    n130 = Greater Or Equal?(x=w69, y=w72) -> (x >= y?=w71:bool)
    "Current set voltage 2450" <- w70
    "Current set voltage 2410" <- w51
  }
